vi "Obtain Promise.vi"(8 "error in (no error)":errorcluster, 9 "create if not found? (T)":bool=TRUE, 11 "name (unnamed)":string) -> (0 "error out":errorcluster, 1 "created new?":bool, 3 "Promise out":refnum<class "Promise.lvclass">)   [LabVIEW 2017, in "Promise Future.lvlib" / "Promise.lvclass"]
uses:
  Promise.lvclass
  E:/Promise/Promise Future/Future/Future.lvclass
  Future/Future.lvclass
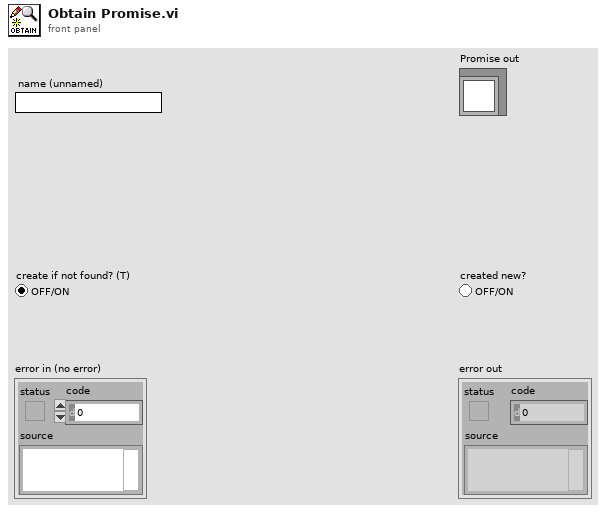
[diagram p1: front panel]
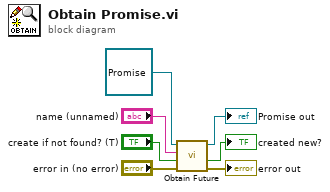
[diagram p0: block diagram]
diagram:
  n1 = call "Obtain Future.vi"("error in (no error)"="error in (no error)", "create if not found? (T)"="create if not found? (T)", "name (unnamed)"="name (unnamed)", "Future in"=refnum<class "Promise.lvclass"> refnum ("Promise Future.lvlib:Promise.lvclass")) -> ("error out"=→"error out":errorcluster, "created new?"=→"created new?":bool, "Future out"=→"Promise out":refnum<class "Promise.lvclass">)  [unwired: 5 in]
